vi "test_CCDSetAndGetSpeed.vi"(7 "Test should pass":bool=TRUE, 8 "error in":errorcluster, 9 "tear down connection":bool=TRUE, 10 "set-up a connection":bool=TRUE, 11 "device selection":enum16{"monochromator", "CCD", "SCD"}(ring)=enum."CCD") -> (0 "error out":errorcluster)   [LabVIEW 2023]
uses:
  Source/Classes/Mono/Monochromator.lvclass
  Source/Classes/CCD/CCD.lvclass
  Source/Classes/SCD/SCD.lvclass
  Source/Classes/CCD/SpeedTokenEnum.ctl
  <vilib>/addons/_JKI Toolkits/Caraya/classes/Assert/Assert Not Error.vi
  <vilib>/addons/_JKI Toolkits/Caraya/classes/Assert/Assert Equal Value and Type_Variant.vi
  Source/Classes/GenericDevice/GenericDevice.lvclass
  <vilib>/addons/_JKI Toolkits/Caraya/classes/Test/Test.lvclass
  <vilib>/addons/_JKI Toolkits/Caraya/classes/Assert/Assert.lvclass
  C:/Users/grju/Desktop/AbgelegteDokumente/Kunden/Horiba/horiba-labview-sdk/Source/Classes/GenericDevice/GenericDevice.lvclass
  C:/Users/grju/Desktop/AbgelegteDokumente/Kunden/Horiba/horiba-labview-sdk/Source/Classes/CCD/CCD.lvclass
panel:
  # "Connector Pane"
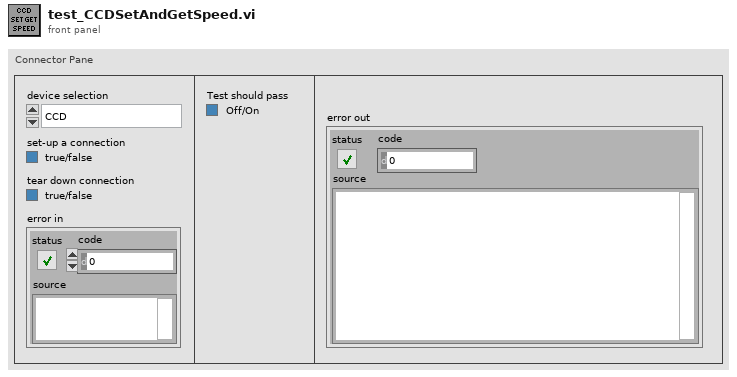
[diagram p1: front panel]
types:
  T1 = typedef "CCD.lvclass/SpeedTokenEnum.ctl" = enum16{"45 kHz       ", " 1 MHz       ", " 1 MHz Ultra "}
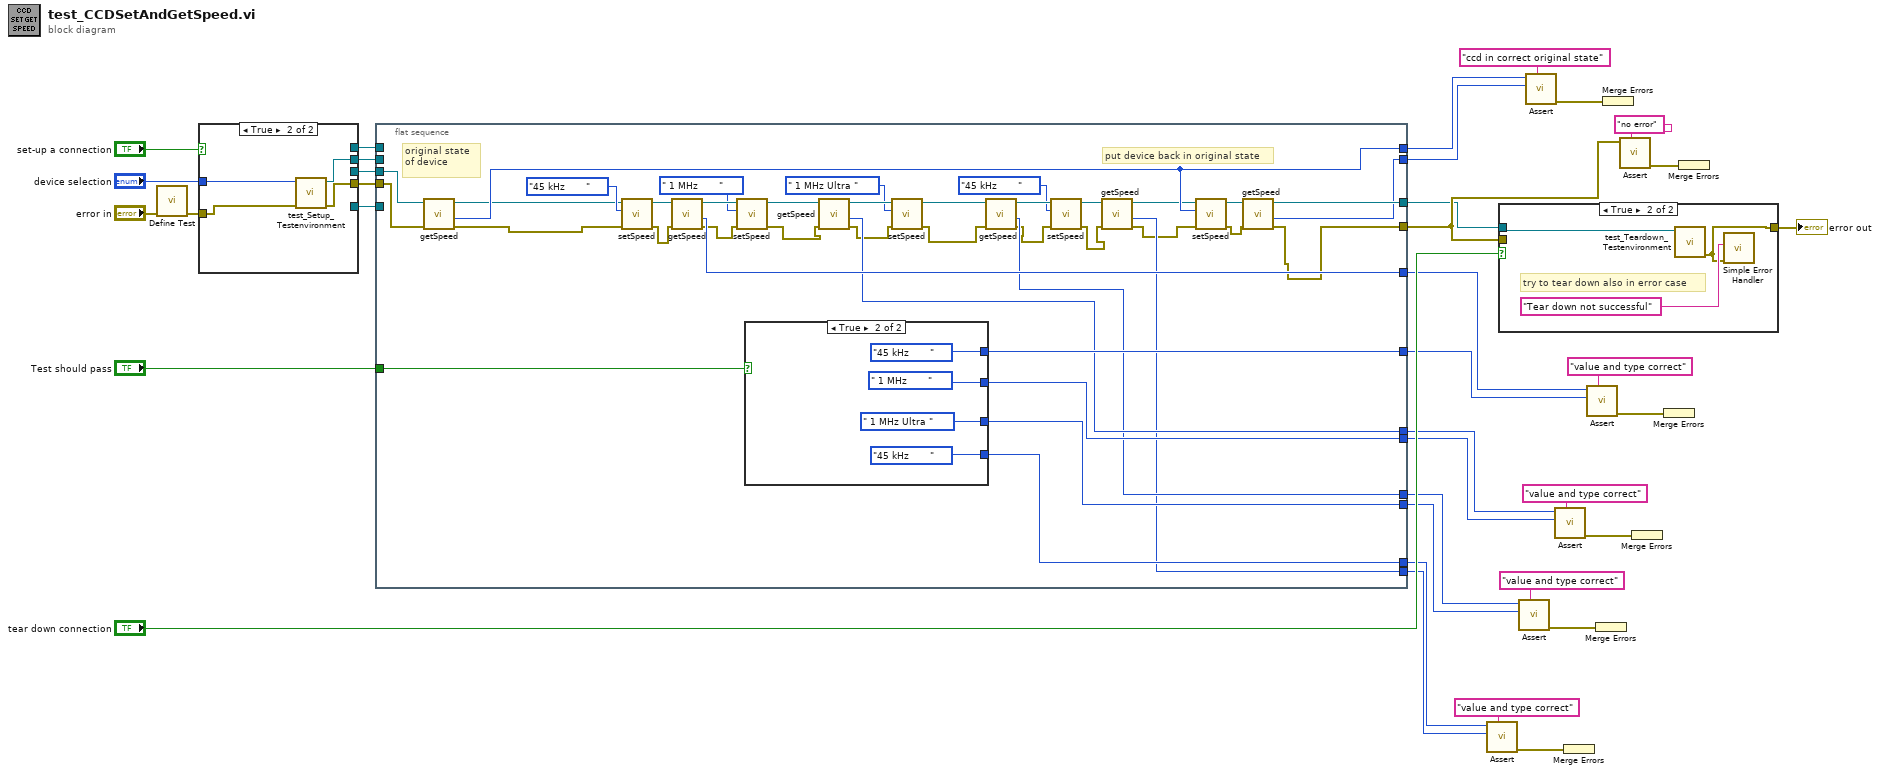
[diagram p0: block diagram]
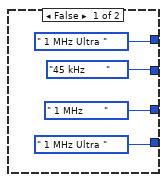
[diagram p2: hidden frame]
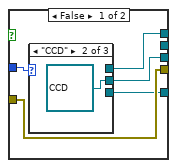
[diagram p3: hidden frame]
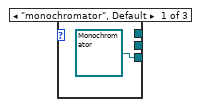
[diagram p4: hidden frame]
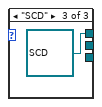
[diagram p5: hidden frame]
diagram:
  n1 = call <vilib>:"Define Test.vi"("error in (no error)"="error in") -> ("error out"=w32:errorcluster)  [unwired: 9 in, 1 out]
  n2 = case shown="True" "set-up a connection" {
    tunnel: w32 -> [w41 w48]
    tunnel: [w41 w47] -> w34
    tunnel: "device selection" -> [w40 w46]
    tunnel: [_ w45] -> w31
    tunnel: [w39 _] -> w30
    tunnel: [w38 _] -> w29
    tunnel: [w37 _] -> w28
    frame False {
      n3 = case shown="\"CCD\"" w40 {
        tunnel: [refnum<class "Monochromator.lvclass"> refnum ("Monochromator.lvclass") _ _] -> w39
        tunnel: [_ refnum<class "CCD.lvclass"> refnum ("CCD in") _] -> w38
        tunnel: [_ _ refnum<class "SCD.lvclass"> refnum ("SCD.lvclass")] -> w37
        frame "monochromator", Default {
        }
        frame "CCD" {
        }
        frame "SCD" {
        }
      }
    }
    frame True {
      n4 = call "test_Setup_Testenvironment.vi"("error in"=w48, "device selection"=w46) -> ("error out"=w47:errorcluster, "GenericDevice.lvclass"=w45:refnum<class "GenericDevice.lvclass">)  [unwired: 7 in, 1 out]
    }
  }
  n5 = flat-sequence {
    tunnel: w34 -> [w81]
    tunnel: w31 -> [_]
    tunnel: w30 -> [_]
    tunnel: w29 -> [w82]
    tunnel: w28 -> [_]
    tunnel: [w59] -> w23
    tunnel: "Test should pass" -> [w87]
    tunnel: [w78] -> w22
    tunnel: [w77] -> w19
    tunnel: [w79] -> w18
    tunnel: [w73] -> w17
    tunnel: [w72] -> w15
    tunnel: [w71] -> w13
    tunnel: [w70] -> w10
    tunnel: [w86] -> w16
    tunnel: [w85] -> w14
    tunnel: [w83] -> w12
    tunnel: [w84] -> w11
    frame #0 {
      # "put device back in original state"
      # "original state of device"
      n6 = call "getSpeed.vi"("error in (no error)"=w81, "CCD in"=w82) -> ("error out"=w49:errorcluster, "speed info (enum)"=w79:T1, "CCD out"=w68:refnum<class "CCD.lvclass">)  [unwired: 6 in, 1 out]
      n7 = call "setSpeed.vi"("error in (no error)"=w49, "speed"=SpeedTokenEnum."45 kHz       ", "CCD in"=w68) -> ("error out"=w50:errorcluster, "CCD out"=w75:refnum<class "CCD.lvclass">)  [unwired: 5 in, 2 out]
      n8 = call "getSpeed.vi"("error in (no error)"=w50, "CCD in"=w75) -> ("error out"=w51:errorcluster, "speed info (enum)"=w73:T1, "CCD out"=w76:refnum<class "CCD.lvclass">)  [unwired: 6 in, 1 out]
      n9 = call "setSpeed.vi"("error in (no error)"=w51, "speed"=SpeedTokenEnum." 1 MHz       ", "CCD in"=w76) -> ("error out"=w52:errorcluster, "CCD out"=w63:refnum<class "CCD.lvclass">)  [unwired: 5 in, 2 out]
      n10 = case shown="True" w87 {
        tunnel: [SpeedTokenEnum." 1 MHz Ultra " ("speed") SpeedTokenEnum."45 kHz       " ("speed")] -> w86
        tunnel: [SpeedTokenEnum."45 kHz       " ("speed") SpeedTokenEnum." 1 MHz       " ("speed")] -> w85
        tunnel: [SpeedTokenEnum." 1 MHz       " ("speed") SpeedTokenEnum." 1 MHz Ultra " ("speed")] -> w83
        tunnel: [SpeedTokenEnum." 1 MHz Ultra " ("speed") SpeedTokenEnum."45 kHz       " ("speed")] -> w84
        frame False {
        }
        frame True {
        }
      }
      n11 = call "getSpeed.vi"("error in (no error)"=w52, "CCD in"=w63) -> ("error out"=w53:errorcluster, "speed info (enum)"=w72:T1, "CCD out"=w67:refnum<class "CCD.lvclass">)  [unwired: 6 in, 1 out]
      n12 = call "setSpeed.vi"("error in (no error)"=w53, "speed"=SpeedTokenEnum." 1 MHz Ultra ", "CCD in"=w67) -> ("error out"=w54:errorcluster, "CCD out"=w66:refnum<class "CCD.lvclass">)  [unwired: 5 in, 2 out]
      n13 = call "getSpeed.vi"("error in (no error)"=w54, "CCD in"=w66) -> ("error out"=w55:errorcluster, "speed info (enum)"=w71:T1, "CCD out"=w65:refnum<class "CCD.lvclass">)  [unwired: 6 in, 1 out]
      n14 = call "setSpeed.vi"("error in (no error)"=w55, "speed"=SpeedTokenEnum."45 kHz       ", "CCD in"=w65) -> ("error out"=w56:errorcluster, "CCD out"=w64:refnum<class "CCD.lvclass">)  [unwired: 5 in, 2 out]
      n15 = call "getSpeed.vi"("error in (no error)"=w56, "CCD in"=w64) -> ("error out"=w57:errorcluster, "speed info (enum)"=w70:T1, "CCD out"=w69:refnum<class "CCD.lvclass">)  [unwired: 6 in, 1 out]
      n16 = call "setSpeed.vi"("error in (no error)"=w57, "speed"=w79, "CCD in"=w69) -> ("error out"=w58:errorcluster, "CCD out"=w80:refnum<class "CCD.lvclass">)  [unwired: 5 in, 2 out]
      n17 = call "getSpeed.vi"("error in (no error)"=w58, "CCD in"=w80) -> ("error out"=w59:errorcluster, "speed info (enum)"=w77:T1, "CCD out"=w78:refnum<class "CCD.lvclass">)  [unwired: 6 in, 1 out]
    }
  }
  n18 = call-poly <vilib>:"Assert.vi"("Label"="value and type correct" ("Label (VI Title)"), "Y"=w10, "X"=w11) -> ("error out"=w3:errorcluster)  [unwired: 7 in, 1 out]
  n19 = case shown="True" "tear down connection" {
    tunnel: w22 -> [_ w98]
    tunnel: [w96 w97] -> w1
    tunnel: w23 -> [w96 _]
    frame False {
    }
    frame True {
      # "try to tear down also in error case"
      n20 = call "test_Teardown_Testenvironment.vi"("GenericDevice.lvclass"=w98) -> ("error out"=w97:errorcluster)  [unwired: 9 in, 1 out]
      n21 = call <vilib>:"Simple Error Handler.vi"("error source (\" \")"="Tear down not successful" ("error source (\" \")"), "error in (no error)"=w97) -> ()  [unwired: 3 in, 5 out]
    }
  }
  "error out" <- w1
  n22 = call-poly <vilib>:"Assert.vi"("Label"="value and type correct" ("Label (VI Title)"), "Y"=w12, "X"=w13) -> ("error out"=w2:errorcluster)  [unwired: 7 in, 1 out]
  n23 = call-poly <vilib>:"Assert.vi"("Label"="ccd in correct original state" ("Label (VI Title)"), "Y"=w19, "X"=w18) -> ("error out"=w21:errorcluster)  [unwired: 7 in, 1 out]
  n24 = call-poly <vilib>:"Assert.vi"("Label"="value and type correct" ("Label (VI Title)"), "Y"=w14, "X"=w15) -> ("error out"=w6:errorcluster)  [unwired: 7 in, 1 out]
  n25 = Merge Errors(w3) -> ()  [unwired: 1 out]
  n26 = call-poly <vilib>:"Assert.vi"("Label"="value and type correct" ("Label (VI Title)"), "Y"=w16, "X"=w17) -> ("error out"=w8:errorcluster)  [unwired: 7 in, 1 out]
  n27 = Merge Errors(w2) -> ()  [unwired: 1 out]
  n28 = Merge Errors(w21) -> ()  [unwired: 1 out]
  n29 = call-poly <vilib>:"Assert.vi"("Label"="no error" ("Label (VI Title)"), "Not Error?"=w23) -> ("error out"=w25:errorcluster)  [unwired: 8 in, 1 out]
  n30 = Merge Errors(w6) -> ()  [unwired: 1 out]
  n31 = Merge Errors(w8) -> ()  [unwired: 1 out]
  n32 = Merge Errors(w25) -> ()  [unwired: 1 out]
